vi "vi-scripting-server.vi"(7 "LabVIEW Web Service Request":refnum<class "Web Request.lvclass">) -> ()   [LabVIEW 2025]
uses:
  <vilib>/wsapi/Web Request.lvclass
  LabVIEW-MCP-Server-Toolkit/src/MCP Server/MCP Server.lvlib
panel:
  # "Use the Web Service Request input terminal to call the VIs on the Web Services palette. Do not remove it from the connector pane unless you don't need access to the palette."
  # "Each additional control wired to the connector pane will be available as an input in the URL. To include an indicator in terminal-mode output (the default setting), it must also be wired to the connector pane."
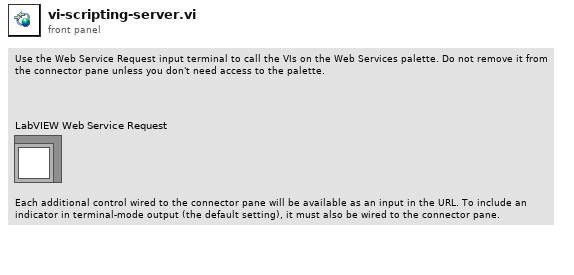
[diagram p1: front panel]
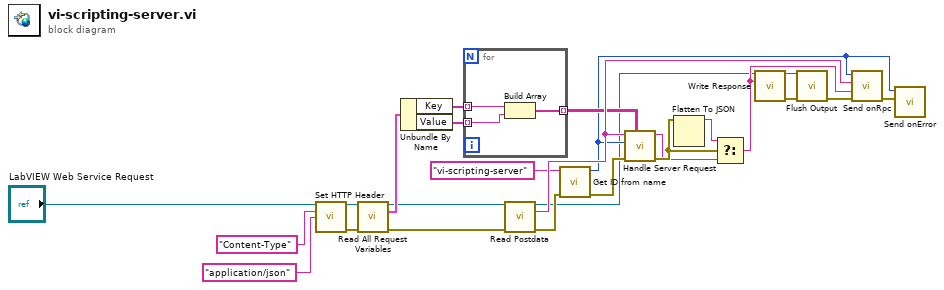
[diagram p0: block diagram]
diagram:
  n1 = call <vilib>:"Set HTTP Header.vi"("LabVIEW Web Service Request"="LabVIEW Web Service Request", "header"="Content-Type", "header value"="application/json") -> ("LabVIEW Web Service Request out"=w21:refnum<class "Web Request.lvclass">, "error out"=w18:errorcluster)  [unwired: 11 in]
  n2 = call <vilib>:"Read All Request Variables.vi"("LabVIEW Web Service Request"=w21, "error in (no error)"=w18) -> ("LabVIEW Web Service Request out"=w14:refnum<class "Web Request.lvclass">, "request variables"=w22:cluster{"Key":string[], "Value":string[]}, "error out"=w13:errorcluster)  [unwired: 11 in]
  n3 = Unbundle By Name(w22) -> ("Key"=w23:string[], "Value"=w24:string[])
  n4 = for {
    tunnel: [w28] -> w15 mode=indexing
    tunnel: w23 -> [w27] mode=indexing
    tunnel: w24 -> [w26] mode=indexing
    n5 = Build Array(w27, w26) -> (w28:string[])
  }
  n6 = call <vilib>:"Read Postdata.vi"("LabVIEW Web Service Request"=w14, "error in (no error)"=w13) -> ("LabVIEW Web Service Request out"=w2:refnum<class "Web Request.lvclass">, "postdata"=w25:string, "error out"=w11:errorcluster)  [unwired: 11 in]
  n7 = call "Get ID from name.vi"("error in (no error)"=w11, "Name"="vi-scripting-server" ("Server Name")) -> ("error out"=w10:errorcluster, "id out"=w4:i32)  [unwired: 7 in, 1 out]
  n8 = call "Handle Server Request.vi"("parameters"=w15, "error in (no error)"=w10, "id in"=w4, "request"=w25) -> ("error out"=w16:errorcluster, "response"=w9:string)  [unwired: 6 in]
  n9 = Flatten To JSON(anything=w16) -> (JSON string=w17:string)  [unwired: 2 in, 1 out]
  n10 = Select(t=w17, s=w16, f=w9) -> (s? t:f=w8:string)
  n11 = call <vilib>:"Write Response.vi"("LabVIEW Web Service Request"=w2, "response string"=w8) -> ("LabVIEW Web Service Request out"=w7:refnum<class "Web Request.lvclass">, "error out"=w6:errorcluster)  [unwired: 12 in]
  n12 = call <vilib>:"Flush Output.vi"("LabVIEW Web Service Request"=w7, "error in (no error)"=w6) -> ("error out"=w5:errorcluster)  [unwired: 12 in, 1 out]
  n13 = call "Send onRpc.vi"("error in (no error)"=w5, "response"=w8, "request"=w25, "id"=w4) -> ("error out"=w3:errorcluster)  [unwired: 7 in]
  n14 = call "Send onError.vi"("error to report"=w3, "id"=w4) -> ()  [unwired: 9 in, 1 out]
